vi "Pivot Drive.vi"(0 "RobotDriveDevRef":T1={"DevStatus"={"status"=FALSE, "code"=0, "source"=""}, "Motors[]"=[], "Square Inputs"=FALSE, "Max Output"=1.0, "Isochronous"=FALSE}, 1 "RobotPivotDevRef":T1={"DevStatus"={"status"=FALSE, "code"=0, "source"=""}, "Motors[]"=[], "Square Inputs"=FALSE, "Max Output"=1.0, "Isochronous"=FALSE}, 3 "Rear Left Current Pivot Angle":dbl, 4 "Rear Right Current Pivot Angle":dbl, 5 "Front Left Current Pivot Angle":dbl, 6 "Front Right Current Pivot Angle":dbl, 7 "error in (no error)":errorcluster, 8 "Rear Left Wanted Pivot Angle":dbl, 9 "Rear Left Speed":dbl, 10 "Rear Right Wanted Pivot Angle":dbl, 11 "Rear Right Speed":dbl, 12 "Front Left Wanted Pivot Angle":dbl, 13 "Front Left Speed":dbl, 14 "Front Right Wanted Pivot Angle":dbl, 15 "Front Right Speed":dbl) -> (20 "RobotDriveDevRef Out":T1={"DevStatus"={"status"=FALSE, "code"=0, "source"=""}, "Motors[]"=[], "Square Inputs"=FALSE, "Max Output"=1.0, "Isochronous"=FALSE}, 21 "RobotPivotDevRef Out":T1={"DevStatus"={"status"=FALSE, "code"=0, "source"=""}, "Motors[]"=[], "Square Inputs"=FALSE, "Max Output"=1.0, "Isochronous"=FALSE}, 27 "error out":errorcluster)   [LabVIEW 2011, in "Pivot Drive.lvlib"]
doc: "Configures the motors for complete control over the pivot drive. This VI allows for controll over every variable in the pivot drive system."
uses:
  Pivot Drive.lvlib
  <vilib>/Rock Robotics/WPI/RobotDrive/WPI_RobotDriveDevRef.ctl
  <vilib>/Rock Robotics/WPI/MotorControl/WPI_MotorControlDeviceRef.ctl
  <vilib>/Rock Robotics/SystemInterfaces/Typedef/FPGA_TypedefDigitalModule.ctl
  <vilib>/Rock Robotics/SystemInterfaces/DIO/FPGA_DIOPWMChannel.ctl
  <vilib>/Rock Robotics/WPI/PWM/WPI_PWMDeadband.ctl
  <vilib>/Rock Robotics/WPI/CAN/Jaguar/SubVIs/WPI_CANJaguar_ControlMode.ctl
  <vilib>/Rock Robotics/WPI/PWM/WPI_PWMTransform_ConPane.ctl
  <vilib>/Rock Robotics/WPI/RobotDrive/WPI_RobotDriveMotorSelectorEnum.ctl
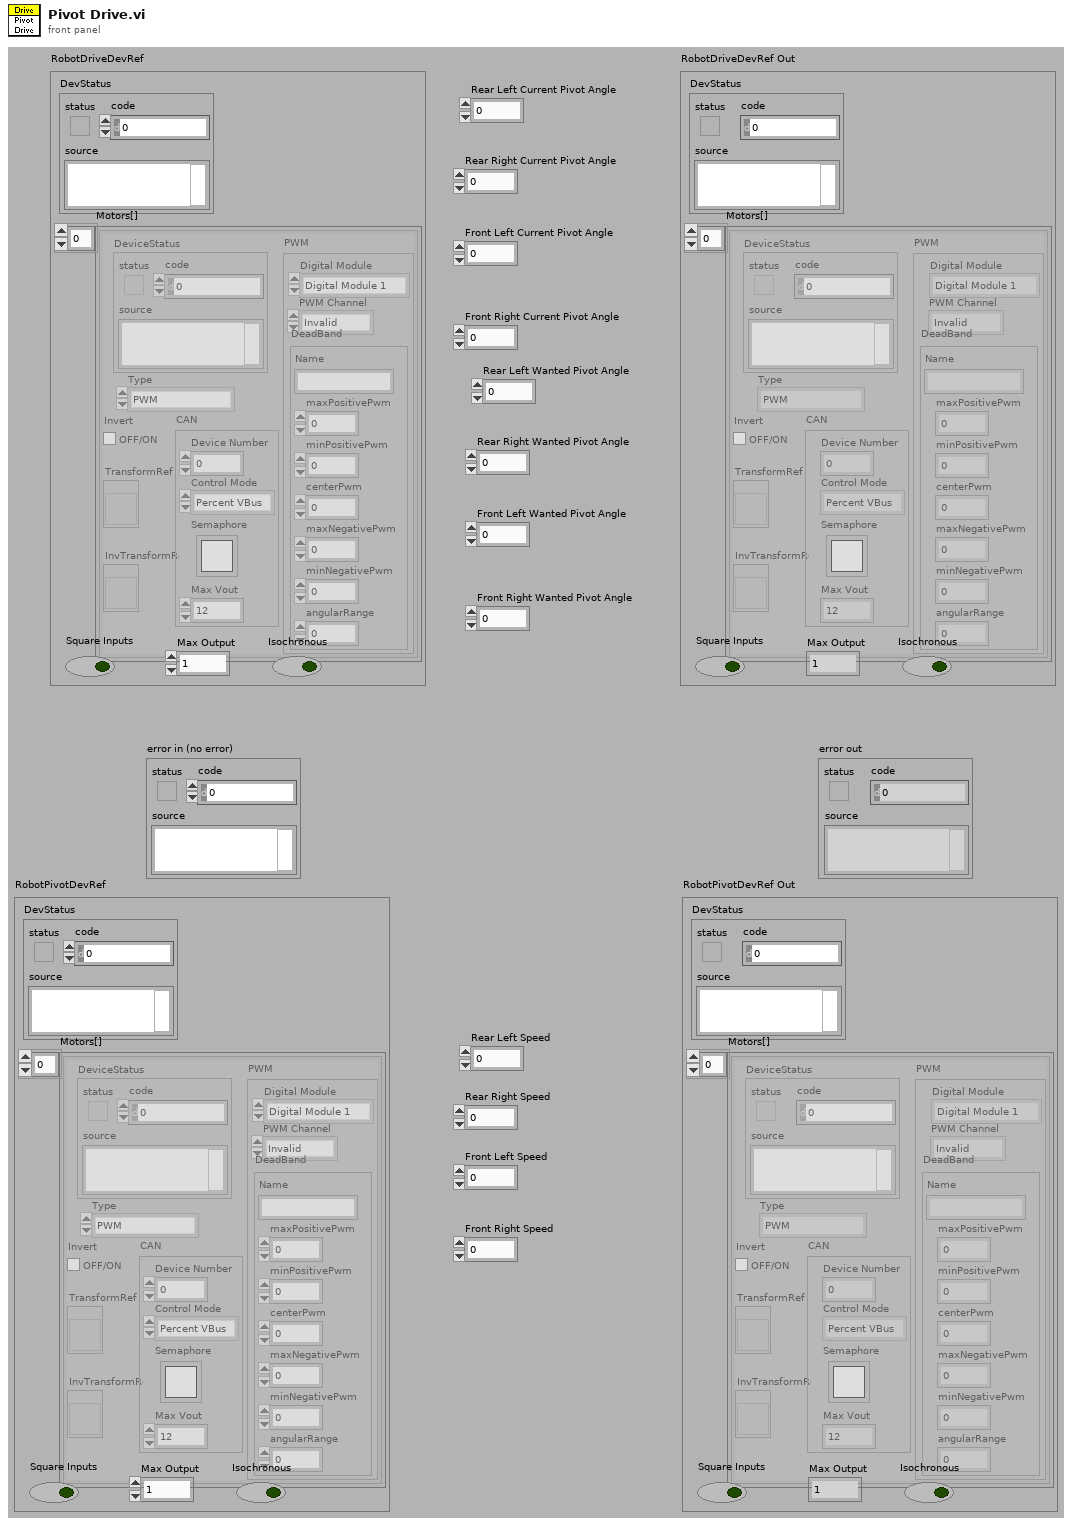
[diagram p1: front panel]
types:
  T1 = typedef "WPI_RobotDriveDevRef.ctl" = cluster{"DevStatus":errorcluster, "Motors[]":T2[], "Square Inputs":bool, "Max Output":dbl, "Isochronous":bool}
  T2 = typedef "WPI_MotorControlDeviceRef.ctl" = cluster{"DeviceStatus":errorcluster, "Type":enum16{"PWM", "CAN"}, "PWM":cluster{"Digital Module":T3, "PWM Channel":T4, "DeadBand":T5}, "CAN":cluster{"Device Number":u8, "Control Mode":T6, "Semaphore":T7, "Max Vout":dbl}, "Invert":bool, "TransformRef":T8, "InvTransformRef":T8}
  T3 = typedef "FPGA_TypedefDigitalModule.ctl" = enum16{"Digital Module 1", "Digital Module 2"}
  T4 = typedef "FPGA_DIOPWMChannel.ctl" = enum8{"PWM 1", "PWM 2", "PWM 3", "PWM 4", "PWM 5", "PWM 6", "PWM 7", "PWM 8", "PWM 9", "PWM 10", "Invalid"}
  T5 = typedef "WPI_PWMDeadband.ctl" = cluster{"Name":string, "maxPositivePwm":i32, "minPositivePwm":i32, "centerPwm":i32, "maxNegativePwm":i32, "minNegativePwm":i32, "angularRange":u16}
  T6 = typedef "WPI_CANJaguar_ControlMode.ctl" = enum8{"Percent VBus", "Current", "Speed", "Position", "Voltage"}
  T7 = typedef "Semaphore RefNum" = refnum<k1>
  T8 = typedef "WPI_PWMTransform_ConPane.ctl" = refnum<vi>
  T9 = cluster{"proportional gain (Kc)":dbl, "integral time (Ti, min)":dbl, "derivative time (Td, min)":dbl}
  T10 = typedef "WPI_RobotDriveMotorSelectorEnum.ctl" = enum16{"Rear Left Motor", "Rear Right Motor", "Front Left Motor", "Front Right Motor"}
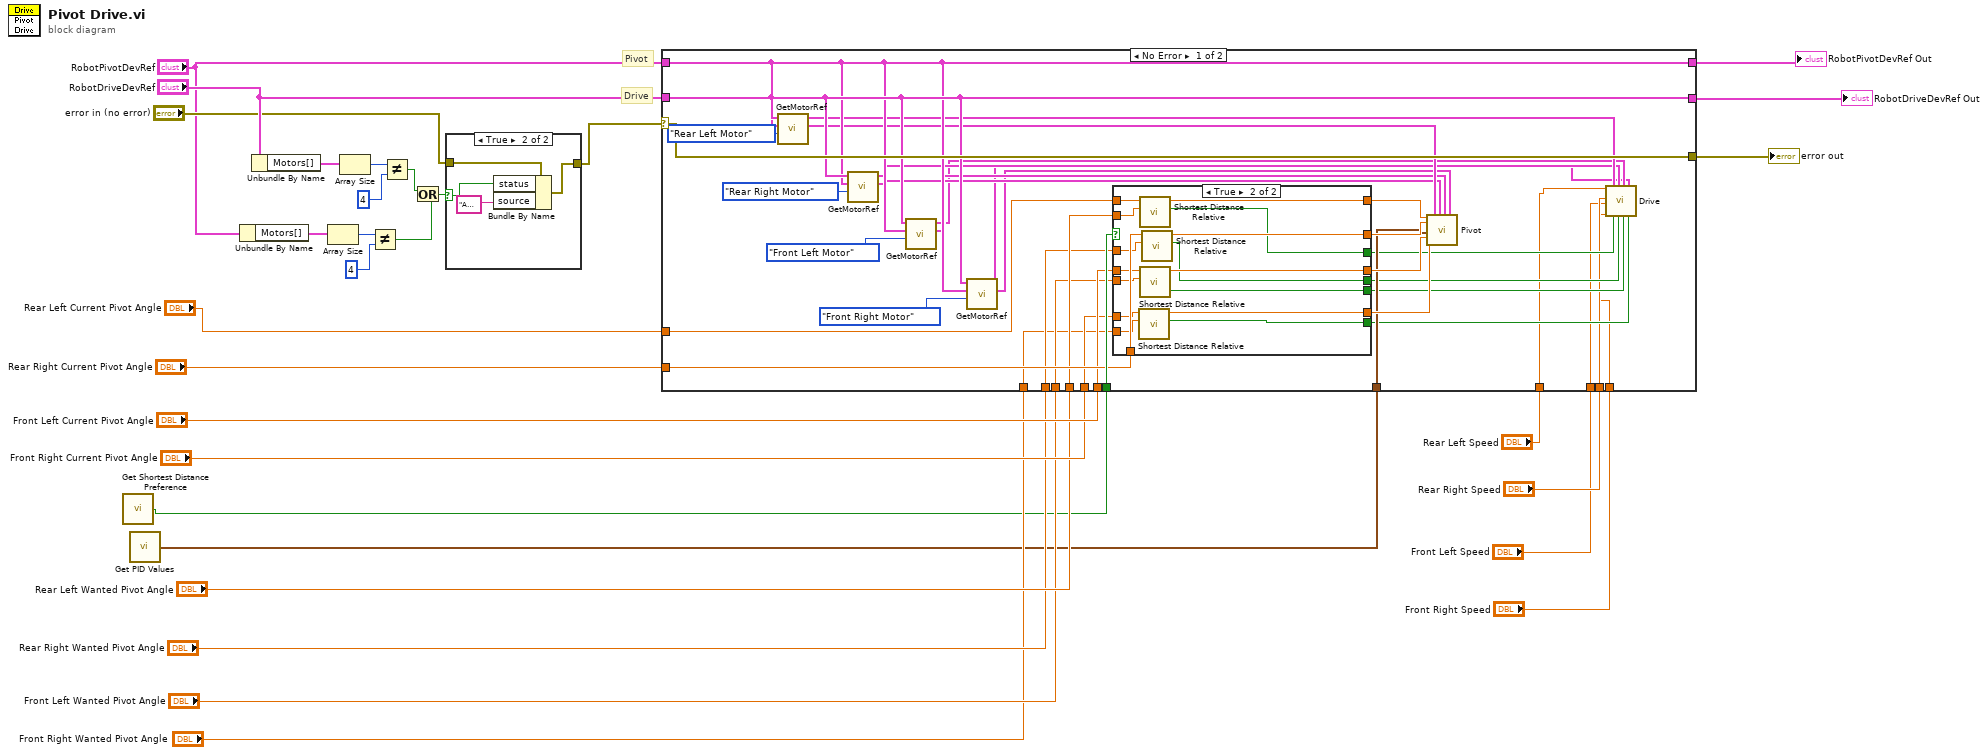
[diagram p0: block diagram]
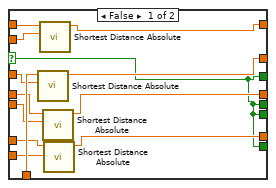
[diagram p3: hidden frame]
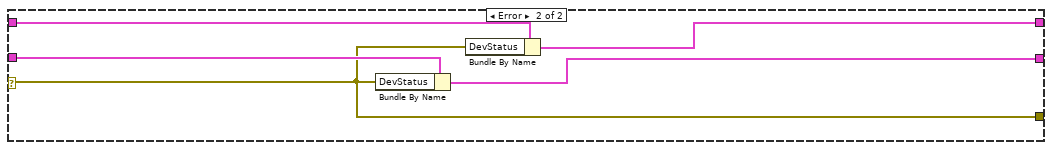
[diagram p4: hidden frame]
diagram:
  # "Drive"
  # "Pivot"
  n1 = call "Get Shortest Distance Preference.vi"() -> ("Use Shortest Distance Relative? Out"=w1:bool)
  n2 = call "Get PID Values.vi"() -> ("PID gains Out"=w2:T9)
  n3 = Unbundle By Name("RobotPivotDevRef") -> ("Motors[]"=w20:T2[])
  n4 = Unbundle By Name("RobotDriveDevRef") -> ("Motors[]"=w28:T2[])
  n5 = Array Size(array=w20) -> (size(s)=w19:i32)
  n6 = Array Size(array=w28) -> (size(s)=w27:i32)
  n7 = Not Equal?(x=w19, y=4) -> (x != y?=w17:bool)
  n8 = Not Equal?(x=w27, y=4) -> (x != y?=w21:bool)
  n9 = Or(x=w21, y=w17) -> (x .or. y?=w22:bool)
  n10 = case shown="True" w22 {
    selector: w22 -> [_ w33]
    tunnel: "error in (no error)" -> [w31 w35]
    tunnel: [w31 w34] -> w23
    frame False {
    }
    frame True {
      n11 = Bundle By Name(cluster=w35, "status"=w33, "source"="A Motor Device Reference was more or less than 4 motors in Pivot Drive.vi") -> (w34:errorcluster)
    }
  }
  n12 = case shown="No Error" w23 {
    selector: w23 -> [w72 w103]
    tunnel: [w67 w105] -> w30
    tunnel: "RobotDriveDevRef" -> [w67 w106]
    tunnel: [w72 w103] -> w29
    tunnel: "RobotPivotDevRef" -> [w66 w104]
    tunnel: [w66 w102] -> w15
    tunnel: w1 -> [w65 _]
    tunnel: "Rear Left Current Pivot Angle" -> [w64 _]
    tunnel: "Rear Right Current Pivot Angle" -> [w63 _]
    tunnel: "Front Left Current Pivot Angle" -> [w62 _]
    tunnel: "Front Right Current Pivot Angle" -> [w61 _]
    tunnel: "Rear Left Wanted Pivot Angle" -> [w60 _]
    tunnel: "Rear Right Wanted Pivot Angle" -> [w59 _]
    tunnel: "Front Left Wanted Pivot Angle" -> [w58 _]
    tunnel: "Front Right Wanted Pivot Angle" -> [w57 _]
    tunnel: w2 -> [w52 _]
    tunnel: "Rear Left Speed" -> [w43 _]
    tunnel: "Rear Right Speed" -> [w42 _]
    tunnel: "Front Left Speed" -> [w41 _]
    tunnel: "Front Right Speed" -> [w40 _]
    frame No Error {
      n13 = call "GetMotorRef.vi"("Motor Selector Enum"=WPI_RobotDriveMotorSelectorEnum."Rear Left Motor", "RobotPivotDevRef"=w66, "RobotDriveDevRef"=w67) -> ("PivotMotorControlDeviceRef"=w51:T2, "DriveMotorControlDeviceRef"=w39:T2)  [unwired: 7 out]
      n14 = call "GetMotorRef.vi"("Motor Selector Enum"=WPI_RobotDriveMotorSelectorEnum."Rear Right Motor", "RobotPivotDevRef"=w66, "RobotDriveDevRef"=w67) -> ("PivotMotorControlDeviceRef"=w50:T2, "DriveMotorControlDeviceRef"=w38:T2)  [unwired: 7 out]
      n15 = call "GetMotorRef.vi"("Motor Selector Enum"=WPI_RobotDriveMotorSelectorEnum."Front Left Motor", "RobotPivotDevRef"=w66, "RobotDriveDevRef"=w67) -> ("PivotMotorControlDeviceRef"=w49:T2, "DriveMotorControlDeviceRef"=w37:T2)  [unwired: 7 out]
      n16 = call "GetMotorRef.vi"("Motor Selector Enum"=WPI_RobotDriveMotorSelectorEnum."Front Right Motor", "RobotPivotDevRef"=w66, "RobotDriveDevRef"=w67) -> ("PivotMotorControlDeviceRef"=w48:T2, "DriveMotorControlDeviceRef"=w36:T2)  [unwired: 7 out]
      n17 = case shown="True" w65 {
        selector: w65 -> [w73 _]
        tunnel: w64 -> [w85 w101]
        tunnel: w63 -> [w82 w100]
        tunnel: w62 -> [w79 w99]
        tunnel: w61 -> [w75 w98]
        tunnel: w60 -> [w84 w97]
        tunnel: w59 -> [w81 w96]
        tunnel: w58 -> [w78 w95]
        tunnel: w57 -> [w76 w94]
        tunnel: [w83 w93] -> w56
        tunnel: [w80 w92] -> w55
        tunnel: [w77 w91] -> w54
        tunnel: [w74 w90] -> w53
        tunnel: [w73 w89] -> w47
        tunnel: [w73 w88] -> w46
        tunnel: [w73 w87] -> w45
        tunnel: [w73 w86] -> w44
        frame False {
          n18 = call "Shortest Distance Absolute.vi"("Set point"=w81, "Current Angle"=w82) -> ("Degres To Travel"=w80:dbl)  [unwired: 9 out]
          n19 = call "Shortest Distance Absolute.vi"("Set point"=w84, "Current Angle"=w85) -> ("Degres To Travel"=w83:dbl)  [unwired: 9 out]
          n20 = call "Shortest Distance Absolute.vi"("Set point"=w78, "Current Angle"=w79) -> ("Degres To Travel"=w77:dbl)  [unwired: 9 out]
          n21 = call "Shortest Distance Absolute.vi"("Set point"=w76, "Current Angle"=w75) -> ("Degres To Travel"=w74:dbl)  [unwired: 9 out]
        }
        frame True {
          n22 = call "Shortest Distance Relative.vi"("Needed angle"=w94, "Current Angle"=w98) -> ("Flip motors?"=w86:bool, "Degrees to travel"=w90:dbl)  [unwired: 8 out]
          n23 = call "Shortest Distance Relative.vi"("Needed angle"=w97, "Current Angle"=w101) -> ("Flip motors?"=w89:bool, "Degrees to travel"=w93:dbl)  [unwired: 8 out]
          n24 = call "Shortest Distance Relative.vi"("Needed angle"=w95, "Current Angle"=w99) -> ("Flip motors?"=w87:bool, "Degrees to travel"=w91:dbl)  [unwired: 8 out]
          n25 = call "Shortest Distance Relative.vi"("Needed angle"=w96, "Current Angle"=w100) -> ("Flip motors?"=w88:bool, "Degrees to travel"=w92:dbl)  [unwired: 8 out]
        }
      }
      n26 = call "Pivot.vi"("Displacement Angle 1"=w56, "Displacement Angle 2"=w55, "PID gains"=w52, "Displacement Angle 3"=w54, "Displacement Angle 4"=w53, "MotorControlDevRef RL"=w51, "MotorControlDevRef RR"=w50, "MotorControlDevRef FL"=w49, "MotorControlDevRef FR"=w48) -> ()  [unwired: 4 in, 7 out]
      n27 = call "Drive.vi"("Drive Motor RL"=w43, "Drive Motor RR"=w42, "Drive Motor FL"=w41, "Drive Motor FR"=w40, "MotorControlDevRef RL"=w39, "Flip Drive Motor RL"=w47, "MotorControlDevRef RR"=w38, "Flip Drive Motor RR"=w46, "MotorControlDevRef FL"=w37, "Flip Drive Motor FL"=w45, "MotorControlDevRef FR"=w36, "Flip Drive Motor FR"=w44) -> ()  [unwired: 8 out]
    }
    frame Error {
      n28 = Bundle By Name(cluster=w106, "DevStatus"=w103) -> (w105:T1)
      n29 = Bundle By Name(cluster=w104, "DevStatus"=w103) -> (w102:T1)
    }
  }
  "RobotDriveDevRef Out" <- w30
  "error out" <- w29
  "RobotPivotDevRef Out" <- w15
